vi "test - TMO of Sync-Reply.vi"(8 "error in (no error)":errorcluster, 11 "TestCase in":refnum<class "testcase-Basic-Function.lvclass">) -> (0 "error out":errorcluster, 3 "TestCase out":refnum<class "testcase-Basic-Function.lvclass">)   [LabVIEW 2017, in "testcase-Basic-Function.lvclass"]
uses:
  testcase-Basic-Function.lvclass
  src/user.lib/_NEVSTOP/Communicable State Machine(CSM)/AdvanceAPI/CSM - Revert Arguments-Safe String.vi
  src/user.lib/_NEVSTOP/Communicable State Machine(CSM)/AdvanceAPI/CSM - Make String Arguments Safe.vi
  src/user.lib/_NEVSTOP/Communicable State Machine(CSM)/AdvanceAPI/CSM - Break Down Multiple States String.vi
  src/user.lib/_NEVSTOP/Communicable State Machine(CSM)/AdvanceAPI/CSM - Compact Multiple States.vi
  src/user.lib/_NEVSTOP/Communicable State Machine(CSM)/AdvanceAPI/CSM - Keywords.vi
  src/user.lib/_NEVSTOP/Communicable State Machine(CSM)/_Shared/Trim Single-line Text.vi
  <vilib>/addons/_JKI Toolkits/VI Tester/TestCase.llb/TestCase.lvclass
  src/user.lib/_NEVSTOP/Communicable State Machine(CSM)/Communicable State Machine.lvlib
  C:/Program Files (x86)/National Instruments/LabVIEW 2017/vi.lib/addons/_JKI Toolkits/VI Tester/TestCase.llb/TestCase.lvclass
panel:
  out "x-y":u32
  out "State History":string
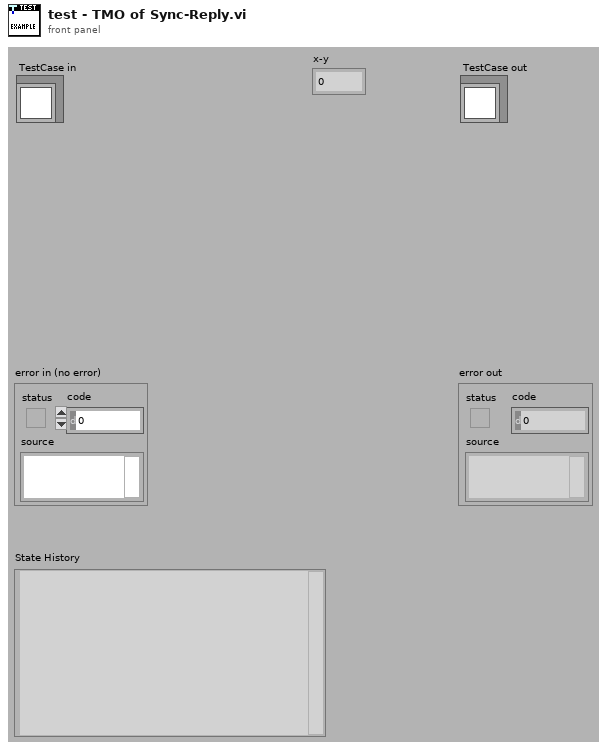
[diagram p1: front panel]
types:
  T1 = enum32{"Invalid", "Standard", "Closed", "Hidden", "Minimized", "Maximized"}
  T2 = enum32{"invalid app kind", "Development System", "Run Time System", "Student Edition", "Embedded LabVIEW", "Evaluation", "Custom"}
  T3 = typedef "Communicable State Machine.lvlib/_CSM_Response Source Message.ctl" = cluster{"‘State":string, "’Arguments":string, "’Error":errorcluster}
  T4 = cluster{"Current VI Reference":refnum<vi>, "Close Panel on Exit?":bool}
  T5 = cluster{"Core":cluster{"Current VI Reference":refnum<vi>, "Close Panel on Exit?":bool}, "Your Boolean data":bool, "Your string data":string}
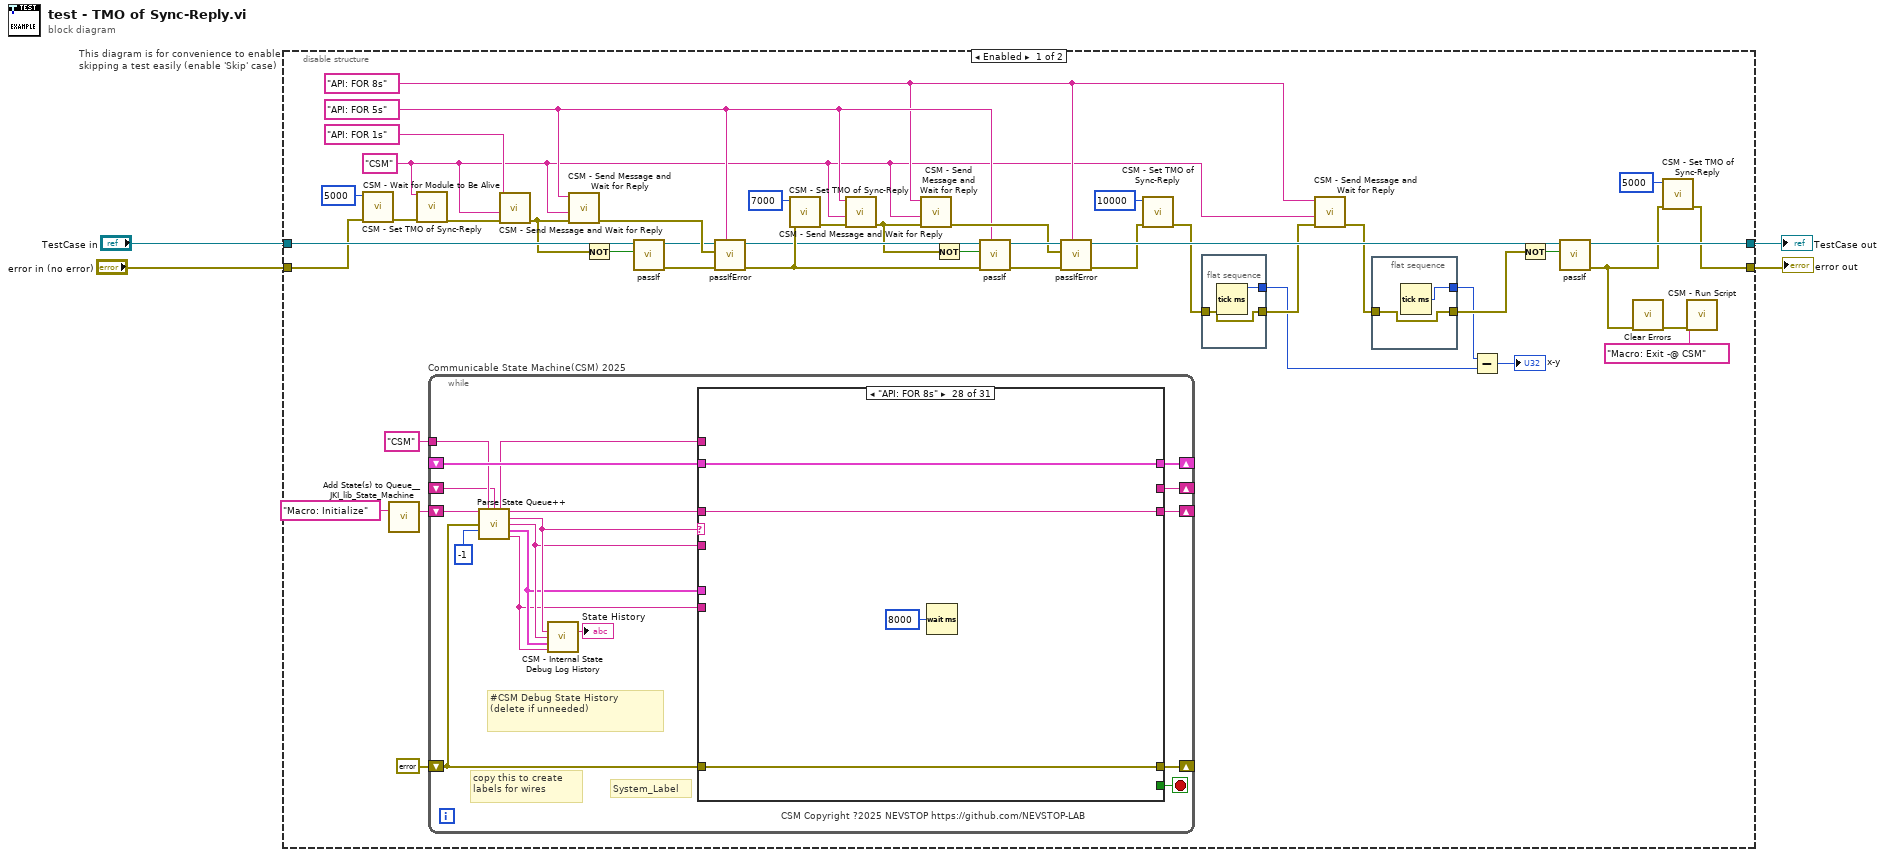
[diagram p0: block diagram]
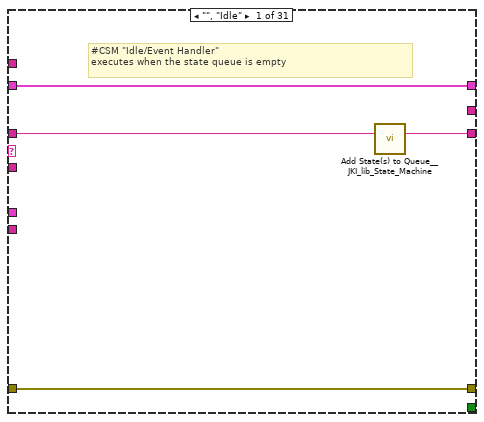
[diagram p2: hidden frame]
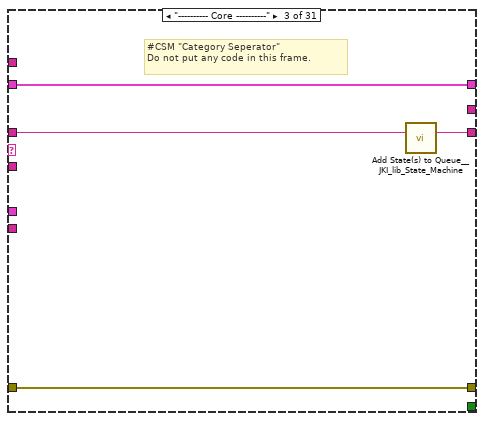
[diagram p4: hidden frame]
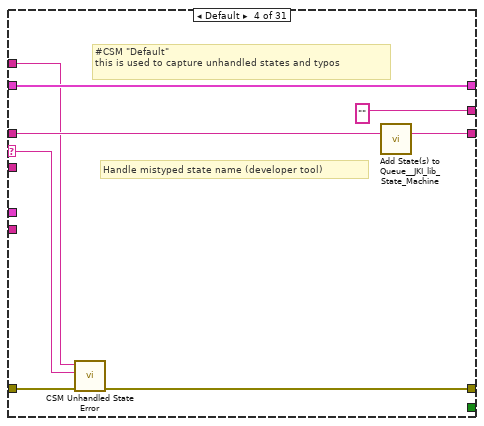
[diagram p5: hidden frame]
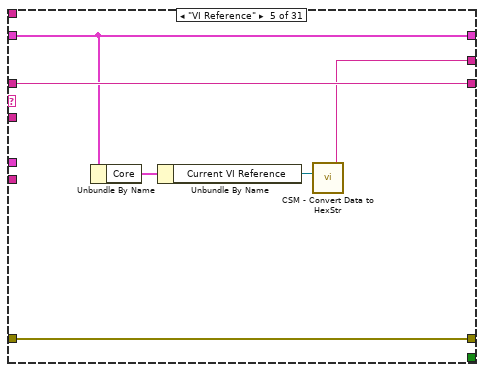
[diagram p6: hidden frame]
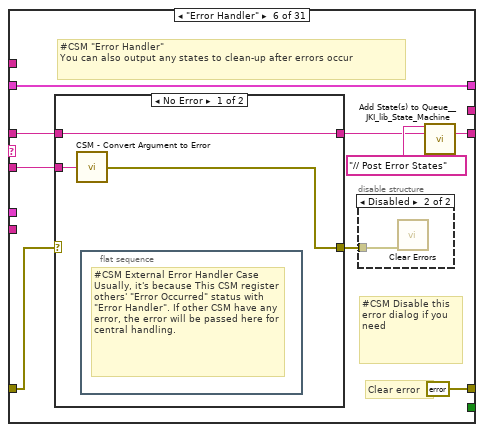
[diagram p7: hidden frame]
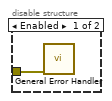
[diagram p8: hidden frame]
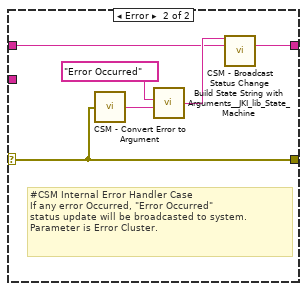
[diagram p9: hidden frame]
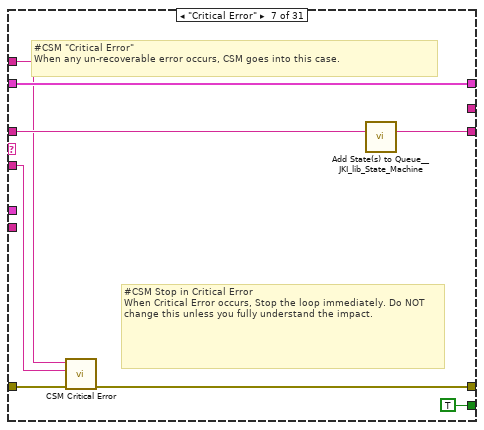
[diagram p10: hidden frame]
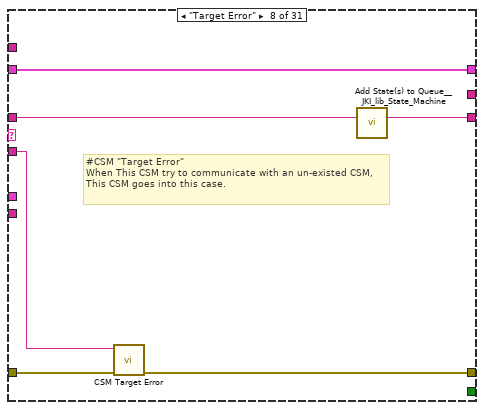
[diagram p11: hidden frame]
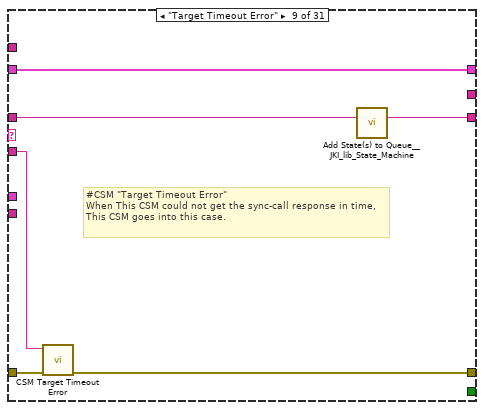
[diagram p12: hidden frame]
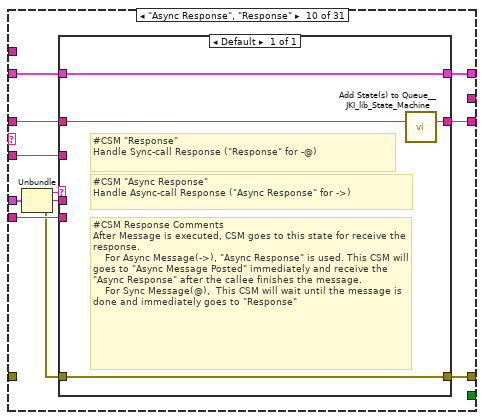
[diagram p13: hidden frame]
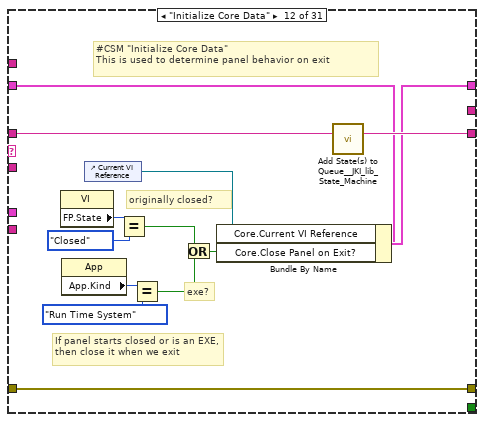
[diagram p15: hidden frame]
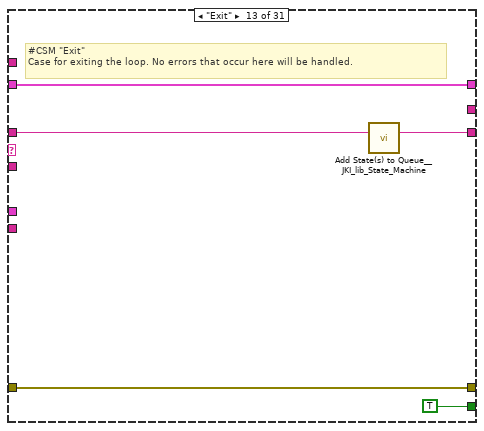
[diagram p16: hidden frame]
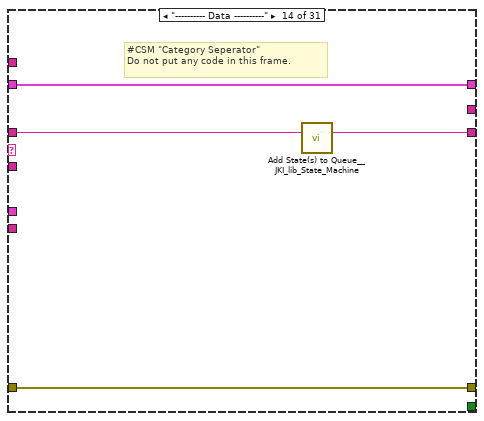
[diagram p17: hidden frame]
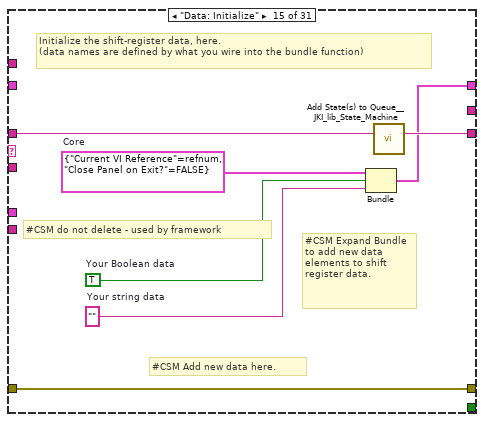
[diagram p18: hidden frame]
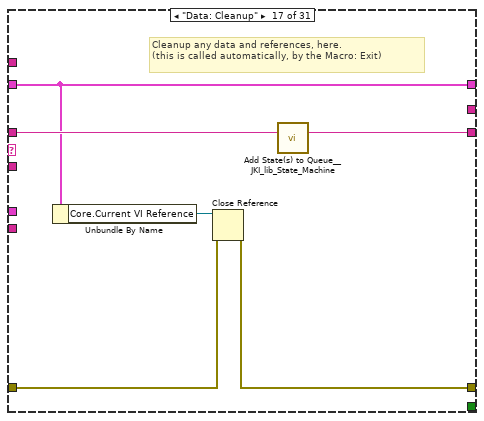
[diagram p20: hidden frame]
diagram:
  n1 = disable-structure "This diagram is for convenience to enable skipping a test easily (enable 'Skip' case)" shown="Enabled" {
    disable-tunnel: "TestCase in" -> [w40 w332]
    disable-tunnel: [w21 w330] -> w1
    disable-tunnel: [w5 w331] -> w3
    disable-tunnel: "error in (no error)" -> [w13 w329]
    frame Enabled {
      w23 = "API: FOR 8s" ("State")
      w27 = "API: FOR 5s" ("State")
      w18 = "CSM" ("Name (\"\" to Use UUID)")
      n2 = call "CSM - Set TMO of Sync-Reply.vi"("Error In"=w13, "TMO For Sync-Rep (Ms) In"=5000 ("TMO for Sync-Rep(ms)")) -> ("error out"=w14:errorcluster)  [unwired: 8 in, 1 out]
      n3 = call <vilib>:"Add State(s) to Queue__JKI_lib_State_Machine.vi"("State(s) in (\"\")"="Macro: Initialize" ("Init State(\"Macro: Initialize\")")) -> ("States Out"=w48:string)  [unwired: 14 in]
      n4 = call "CSM - Wait for Module to Be Alive.vi"("CSM Name"=w18, "error in (no error)"=w14) -> ("error out"=w44:errorcluster)  [unwired: 11 in, 2 out]
      n5 = while "Communicable State Machine(CSM) 2025" {
        shift-right: [w65] -> _
        shift-left: _ -> [w64]
        shift-right: [w68] -> _
        shift-left: errorcluster {"status"=FALSE, "code"=0, "source"=""} ("error out") -> [w63]
        shift-right: [w67] -> _
        shift-left: w48 -> [w69]
        tunnel: "CSM" ("Name (\"\" to Use UUID)") -> [w61]
        shift-right: [w62] -> _
        shift-left: _ -> [w55]
        stop <- w66 stop-if-true
        # "#CSM Debug State History\n(delete if unneeded)"
        # "copy this to create labels for wires"
        # "System_Label"
        # "CSM Copyright ?2025 NEVSTOP https://github.com/NEVSTOP-LAB"
        n6 = call "Parse State Queue++.vi"("State Queue"=w69, "Name (\"\" to Use UUID)"=w61, "Response Arguments"=w55, "Previous Error"=w63, "Dequeue Timeout (1 ms)"=-1 ("Timeout")) -> ("Name Used"=w56:string, "Remaining States"=w70:string, "Current State"=w60:string, "Arguments"=w59:string, ">> Response Source Message >>"=w58:T3, ">> Source CSM >>"=w57:string)  [unwired: 5 in]
        n7 = call "CSM - Internal State Debug Log History.vi"("State"=w60, "Arguments (\"\")"=w59, ">> Response Source Message >>"=w58, "Source (\"\")"=w57) -> ("Debug Log"=→"State History":string)  [unwired: 11 in]
        n8 = case shown="\"API: FOR 8s\"" w60 {
          selector: w60 -> [_ _ _ w84 _ _ _ _ _ _ _ _ _ _ _ _ _ _ _ _ _ _ _ _ _ _ _ _ _ _ _]
          tunnel: w70 -> [w71 w76 w81 w88 w94 w100 w121 w127 w133 w141 w152 w166 w171 w175 w182 w184 w191 w195 w199 w205 w220 w289 w294 w301 w303 w307 w311 w315 w320 w324 w328]
          tunnel: w59 -> [_ _ _ _ _ w99 w117 w126 w131 w140 _ _ _ _ _ _ _ _ _ w200 w214 _ _ _ _ _ _ _ _ _ _]
          tunnel: w64 -> [w72 w75 w78 w86 w93 w103 w122 w128 w134 w143 w151 w159 w169 w172 _ w183 w186 w192 w197 w203 w216 w286 w291 w298 w302 w306 w310 w314 w317 w321 w325]
          tunnel: [w73 w77 w79 w82 w95 errorcluster {"status"=FALSE, "code"=0, "source"=""} ("error out") w118 w124 w130 w146 w153 w163 w168 w173 w179 w185 w187 w193 w196 w201 w217 w287 w292 w299 w304 w308 w312 w316 w318 w322 w326] -> w68
          tunnel: w63 -> [w73 w77 w79 w89 w95 w101 w123 w125 w132 _ w153 w163 w168 w173 w179 w185 w188 w193 w196 w202 w218 w287 w292 w299 w304 w308 w312 w316 w318 w322 w326]
          tunnel: [w74 w76 w80 w87 w94 w96 w120 w129 w135 w142 w152 w165 w170 w174 w181 w184 w190 w194 w198 w204 w219 w288 w293 w300 w303 w307 w311 w315 w319 w323 w327] -> w67
          tunnel: [_ _ _ _ _ _ TRUE _ _ _ _ _ TRUE _ _ _ _ _ _ _ _ _ _ _ _ _ _ _ _ _ _] -> w66
          tunnel: [w72 w75 w78 w86 w93 w103 w122 w128 w134 w144 w151 w164 w169 w172 w180 w183 w186 w192 w197 w203 w216 w286 w291 w298 w302 w306 w310 w314 w317 w321 w325] -> w65
          tunnel: w57 -> [_ _ _ _ _ _ _ _ _ w138 _ _ _ _ _ _ _ _ _ _ _ _ _ _ _ _ _ _ _ _ _]
          tunnel: w58 -> [_ _ _ _ _ _ _ _ _ w145 _ _ _ _ _ _ _ _ _ _ _ _ _ _ _ _ _ _ _ _ _]
          tunnel: [_ _ _ "" w90 _ _ _ _ _ _ _ _ _ _ _ _ _ _ _ _ _ _ _ _ _ _ _ _ _ _] -> w62
          tunnel: w56 -> [_ _ _ w83 _ _ w116 _ _ _ _ _ _ _ _ _ _ _ _ _ _ _ _ _ _ _ _ _ _ _ _]
          frame "", "Idle" {
            # "#CSM \"Idle/Event Handler\"\nexecutes when the state queue is empty"
            n9 = call <vilib>:"Add State(s) to Queue__JKI_lib_State_Machine.vi"("State(s) in (\"\")"=w71) -> ("States Out"=w74:string)  [unwired: 14 in]
          }
          frame "CSM Documentation" {
            # "#CSM README FIRST\n\nCommunicable State Machine(CSM) is a LabVIEW application framework that builds upon JKI State Machine(JKISM). It follows the pattern of JKISM and extends the keywords to describe message communication between modules, including concepts such as Sync-Message, Async-Message, Subscription/Unsubscription of status - essential elements for creating reusable code modules. For more information, please visit the CSM wiki: https://nevstop-lab.github.io/CSM-Wiki/\n\nFor instructions on JKI State Machine, visit: http://jki.net/state-machine/\nFor information about CSM, visit: https://github.com/NEVSTOP-LAB"
            # "#CSM \"Documentation\"\nCase for holding CSM Documenation"
          }
          frame "---------- Core ----------" {
            # "#CSM \"Category Seperator\"\nDo not put any code in this frame."
            n10 = call <vilib>:"Add State(s) to Queue__JKI_lib_State_Machine.vi"("State(s) in (\"\")"=w81) -> ("States Out"=w80:string)  [unwired: 14 in]
          }
          frame Default {
            # "#CSM \"Default\"\nthis is used to capture unhandled states and typos"
            # "Handle mistyped state name (developer tool)"
            n11 = call "CSM Unhandled State Error.vi"("error in (no error)"=w89, "Current State"=w84, "CSM Name"=w83) -> ("error out"=w82:errorcluster)  [unwired: 8 in]
            n12 = call <vilib>:"Add State(s) to Queue__JKI_lib_State_Machine.vi"("State(s) in (\"\")"=w88) -> ("States Out"=w87:string)  [unwired: 14 in]
          }
          frame "VI Reference" {
            n13 = Unbundle By Name(w93) -> ("Core"=w92:T4)
            n14 = Unbundle By Name(w92) -> ("Current VI Reference"=w91:refnum<vi>)
            n15 = call "CSM - Convert Data to HexStr.vi"("Variant"=w91) -> ("HEX String (0-9,A-F)"=w90:string)  [unwired: 8 in]
          }
          frame "Error Handler" {
            # "#CSM Disable this error dialog if you need"
            # "#CSM \"Error Handler\"\nYou can also output any states to clean-up after errors occur"
            # "Clear error"
            n16 = case shown="No Error" w101 {
              selector: w101 -> [_ w110]
              tunnel: [w109 w112] -> w97
              tunnel: w100 -> [w109 w111]
              tunnel: w99 -> [w108 _]
              tunnel: [w107 w110] -> w102
              frame No Error {
                n17 = call "CSM - Convert Argument to Error.vi"("Argument"=w108) -> ("Error"=w107:errorcluster)  [unwired: 4 in]
                n18 = flat-sequence {
                  frame #0 {
                    # "#CSM External Error Handler Case\nUsually, it's because This CSM register others' \"Error Occurred\" status with \"Error Handler\". If other CSM have any error, the error will be passed here for central handling."
                  }
                }
              }
              frame Error {
                # "#CSM Internal Error Handler Case \nIf any error Occurred, \"Error Occurred\" \nstatus update will be broadcasted to system.\nParameter is Error Cluster."
                n19 = call "CSM - Convert Error to Argument.vi"("Error"=w110) -> ("Argument"=w114:string)  [unwired: 4 in]
                n20 = call <vilib>:"Build State String with Arguments__JKI_lib_State_Machine.vi"("Arguments (\"\")"=w114, "State"="Error Occurred" ("Status with Arguments")) -> ("State with Arguments"=w113:string)  [unwired: 4 in]
                n21 = call "CSM - Broadcast Status Change.vi"("Status With Arguments"=w113, "State Queue"=w111) -> ("Remaining States"=w112:string)  [unwired: 13 in]
              }
            }
            n22 = disable-structure shown="Disabled" {
              disable-tunnel: w102 -> [w105 w106]
              frame Enabled {
                n23 = call <vilib>:"General Error Handler.vi"("error in (no error)"=w105) -> ()  [unwired: 10 in, 5 out]
              }
              frame Disabled {
                n24 = call <vilib>:"Clear Errors.vi"("error in (no error)"=w106) -> ()  [unwired: 5 in, 2 out]
              }
            }
            n25 = call <vilib>:"Add State(s) to Queue__JKI_lib_State_Machine.vi"("State(s) in Front (\"\")"="// Post Error States", "State(s) in (\"\")"=w97) -> ("States Out"=w96:string)  [unwired: 13 in]
          }
          frame "Critical Error" {
            # "#CSM Stop in Critical Error\nWhen Critical Error occurs, Stop the loop immediately. Do NOT change this unless you fully understand the impact."
            # "#CSM \"Critical Error\"\nWhen any un-recoverable error occurs, CSM goes into this case."
            n26 = call "CSM Critical Error.vi"("error in (no error)"=w123, "Arugments (As Reason)"=w117, "CSM Name"=w116) -> ("error out"=w118:errorcluster)  [unwired: 8 in]
            n27 = call <vilib>:"Add State(s) to Queue__JKI_lib_State_Machine.vi"("State(s) in (\"\")"=w121) -> ("States Out"=w120:string)  [unwired: 14 in]
          }
          frame "Target Error" {
            # "#CSM \"Target Error\"\nWhen This CSM try to communicate with an un-existed CSM, This CSM goes into this case."
            n28 = call "CSM Target Error.vi"("error in (no error)"=w125, "Arguments (As CSM Name)"=w126) -> ("error out"=w124:errorcluster)  [unwired: 9 in]
            n29 = call <vilib>:"Add State(s) to Queue__JKI_lib_State_Machine.vi"("State(s) in (\"\")"=w127) -> ("States Out"=w129:string)  [unwired: 14 in]
          }
          frame "Target Timeout Error" {
            # "#CSM \"Target Timeout Error\"\nWhen This CSM could not get the sync-call response in time, This CSM goes into this case."
            n30 = call "CSM Target Timeout Error.vi"("error in (no error)"=w132, "Arguments (As CSM Name)"=w131) -> ("error out"=w130:errorcluster)  [unwired: 9 in]
            n31 = call <vilib>:"Add State(s) to Queue__JKI_lib_State_Machine.vi"("State(s) in (\"\")"=w133) -> ("States Out"=w135:string)  [unwired: 14 in]
          }
          frame "Async Response", "Response" {
            n32 = Unbundle(w145) -> ("‘State"=w139:string, "’Arguments"=w137:string, "’Error"=w136:errorcluster)
            n33 = case shown="Default" w139 {
              tunnel: [w150] -> w146
              tunnel: w136 -> [w150]
              tunnel: [w149] -> w144
              tunnel: w143 -> [w149]
              tunnel: [w147] -> w142
              tunnel: w141 -> [w148]
              tunnel: w140 -> [_]
              tunnel: w138 -> [_]
              tunnel: w137 -> [_]
              frame Default {
                # "#CSM Response Comments\nAfter Message is executed, CSM goes to this state for receive the response.\n    For Async Message(->), \"Async Response\" is used. This CSM will goes to \"Async Message Posted\" immediately and receive the \"Async Response\" after the callee finishes the message.\n    For Sync Message(@),  This CSM will wait until the message is done and immediately goes to \"Response\""
                # "#CSM \"Async Response\"\nHandle Async-call Response (\"Async Response\" for ->)"
                # "#CSM \"Response\"\nHandle Sync-call Response (\"Response\" for -@)"
                n34 = call <vilib>:"Add State(s) to Queue__JKI_lib_State_Machine.vi"("State(s) in (\"\")"=w148) -> ("States Out"=w147:string)  [unwired: 14 in]
              }
            }
          }
          frame "Async Message Posted" {
            # "#CSM \"Async Message Posted\"\nAfter Async Message is posted (-> or ->| ), CSM goes to this state for post-action.\nYou can use Argument - State to tell which Async Message is called."
          }
          frame "Initialize Core Data" {
            # "#CSM \"Initialize Core Data\"\nThis is used to determine panel behavior on exit"
            # "originally closed?"
            # "exe?"
            # "If panel starts closed or is an EXE, then close it when we exit"
            n35 = property class="VI"() -> ("FP.State"=w156:T1)  [unwired: 2 in, 2 out]
            n36 = property class="App"() -> ("App.Kind"=w162:T2)  [unwired: 2 in, 2 out]
            n37 = control-ref of="Current VI Reference"() -> (w157:refnum<vi>)
            n38 = Equal?(x=w156, y=T1."Closed" ("Front Panel Window:State")) -> (x = y?=w154:bool)
            n39 = Equal?(x=w162, y=T2."Run Time System" ("Application:Kind")) -> (x = y?=w160:bool)
            n40 = Or(x=w154, y=w160) -> (x .or. y?=w158:bool)
            n41 = Bundle By Name(cluster=w159, "Core.Current VI Reference"=w157, "Core.Close Panel on Exit?"=w158) -> (w164:T5)
            n42 = call <vilib>:"Add State(s) to Queue__JKI_lib_State_Machine.vi"("State(s) in (\"\")"=w166) -> ("States Out"=w165:string)  [unwired: 14 in]
          }
          frame "Exit" {
            # "#CSM \"Exit\"\nCase for exiting the loop. No errors that occur here will be handled."
            n43 = call <vilib>:"Add State(s) to Queue__JKI_lib_State_Machine.vi"("State(s) in (\"\")"=w171) -> ("States Out"=w170:string)  [unwired: 14 in]
          }
          frame "---------- Data ----------" {
            # "#CSM \"Category Seperator\"\nDo not put any code in this frame."
            n44 = call <vilib>:"Add State(s) to Queue__JKI_lib_State_Machine.vi"("State(s) in (\"\")"=w175) -> ("States Out"=w174:string)  [unwired: 14 in]
          }
          frame "Data: Initialize" {
            w176 = T4 {"Current VI Reference"=refnum, "Close Panel on Exit?"=FALSE}  # Core
            w178 = TRUE  # Your Boolean data
            w177 = ""  # Your string data
            # "#CSM do not delete - used by framework"
            # "#CSM Expand Bundle to add new data elements to shift register data."
            # "#CSM Add new data here."
            # "Initialize the shift-register data, here.\n(data names are defined by what you wire into the bundle function)"
            n45 = Bundle("Core"=w176, "Your Boolean data"=w178, "Your string data"=w177) -> (w180:T5)  [unwired: 1 in]
            n46 = call <vilib>:"Add State(s) to Queue__JKI_lib_State_Machine.vi"("State(s) in (\"\")"=w182) -> ("States Out"=w181:string)  [unwired: 14 in]
          }
          frame "Data: Update Indicators" {
          }
          frame "Data: Cleanup" {
            # "Cleanup any data and references, here.\n(this is called automatically, by the Macro: Exit)"
            n47 = Unbundle By Name(w186) -> ("Core.Current VI Reference"=w189:refnum<vi>)
            n48 = Close Reference(reference=w189, error in (no error)=w188) -> (error out=w187:errorcluster)
            n49 = call <vilib>:"Add State(s) to Queue__JKI_lib_State_Machine.vi"("State(s) in (\"\")"=w191) -> ("States Out"=w190:string)  [unwired: 14 in]
          }
          frame "---------- UI ----------" {
            # "#CSM \"Category Seperator\"\nDo not put any code in this frame."
            n50 = call <vilib>:"Add State(s) to Queue__JKI_lib_State_Machine.vi"("State(s) in (\"\")"=w195) -> ("States Out"=w194:string)  [unwired: 14 in]
          }
          frame "UI: Initialize" {
            # "#CSM \"UI: Initialize\"\nInitialize the User Interface, here.\n(this is called automatically, by the Macro: Init)"
            n51 = call <vilib>:"Add State(s) to Queue__JKI_lib_State_Machine.vi"("State(s) in (\"\")"=w199) -> ("States Out"=w198:string)  [unwired: 14 in]
          }
          frame "UI: Cursor Set" {
            # "#CSM \"UI: Cursor Set\"\nSet and Unset Cursor Busy.\n(Usage: \"UI: Cursor Set >> Busy|Idle\")"
            # "Argument"
            n52 = disable-structure shown="TARGET_TYPE!=Windows" {
              disable-tunnel: w202 -> [w208 w213]
              disable-tunnel: [w207 w213] -> w201
              disable-tunnel: w200 -> [w206 _]
              frame condition #0 (active) {
                n53 = case shown="\"Idle\", Default" w206 {
                  tunnel: w208 -> [w210 w212]
                  tunnel: [w209 w211] -> w207
                  frame "Idle", Default {
                    n54 = call <vilib>:"Unset Busy.vi"("error in (no error)"=w210) -> ("error out"=w209:errorcluster)  [unwired: 10 in]
                  }
                  frame "Busy" {
                    n55 = call <vilib>:"Set Busy.vi"("error in (no error)"=w212) -> ("error out"=w211:errorcluster)  [unwired: 9 in, 1 out]
                  }
                }
              }
              frame condition #1 {
              }
            }
            n56 = call <vilib>:"Add State(s) to Queue__JKI_lib_State_Machine.vi"("State(s) in (\"\")"=w205) -> ("States Out"=w204:string)  [unwired: 14 in]
          }
          frame "UI: Front Panel State" {
            # "#CSM \"UI: Front Panel State\"\nSet Front Panel Open or Closed\n(Usage: \"UI: Front Panel State >> Open|Close\")"
            # "Argument"
            n57 = Unbundle By Name(w216) -> ("Core.Current VI Reference"=w215:refnum<vi>)
            n58 = call <vilib>:"Add State(s) to Queue__JKI_lib_State_Machine.vi"("State(s) in (\"\")"=w220) -> ("States Out"=w219:string)  [unwired: 14 in]
            n59 = case shown="\"Close\", \"Closed\"" w214 {
              tunnel: w218 -> [w226 w241 w252 w265 w278]
              tunnel: [w228 w242 w254 w267 w280] -> w217
              tunnel: w215 -> [w227 w239 w253 w266 w279]
              frame "Open", "Standard", Default {
                w221 = T1."Standard" ("State")
                n60 = property class="VI"(reference=w227, error in=w226) -> (reference out=w224:refnum<vi>, error out=w225:errorcluster, "FP.State"=w223:T1)
                n61 = Not Equal?(x=w223, y=w221) -> (x != y?=w222:bool)
                n62 = case shown="True" w222 {
                  tunnel: [w232 w234] -> w228
                  tunnel: w225 -> [w231 w234]
                  tunnel: w224 -> [w230 _]
                  tunnel: w221 -> [w229 _]
                  frame True {
                    n63 = invoke class="VI" method="FP.Open"(reference=w230, error in=w231, "Activate"=TRUE, "State"=w229) -> (error out=w232:errorcluster)  [unwired: 1 in, 4 out]
                  }
                  frame False {
                  }
                }
              }
              frame "Close", "Closed" {
                n64 = property class="VI"(reference=w239, error in=w241) -> (reference out=w238:refnum<vi>, error out=w240:errorcluster, "FP.State"=w236:T1)
                n65 = Not Equal?(x=w236, y=T1."Closed" ("Front Panel Window:State")) -> (x != y?=w235:bool)
                n66 = case shown="False" w235 {
                  tunnel: [w243 w246] -> w242
                  tunnel: w240 -> [w243 w245]
                  tunnel: w238 -> [_ w244]
                  frame False {
                  }
                  frame True {
                    n67 = invoke class="VI" method="FP.Close"(reference=w244, error in=w245) -> (error out=w246:errorcluster)  [unwired: 1 in, 2 out]
                  }
                }
              }
              frame "Hidden", "Hide" {
                w247 = T1."Hidden" ("State")
                n68 = property class="VI"(reference=w253, error in=w252) -> (reference out=w250:refnum<vi>, error out=w251:errorcluster, "FP.State"=w249:T1)
                n69 = Not Equal?(x=w249, y=w247) -> (x != y?=w248:bool)
                n70 = case shown="True" w248 {
                  tunnel: [w258 w259] -> w254
                  tunnel: w251 -> [w257 w259]
                  tunnel: w250 -> [w256 _]
                  tunnel: w247 -> [w255 _]
                  frame True {
                    n71 = invoke class="VI" method="FP.Open"(reference=w256, error in=w257, "State"=w255) -> (error out=w258:errorcluster)  [unwired: 2 in, 4 out]
                  }
                  frame False {
                  }
                }
              }
              frame "Minimize", "Minimized" {
                w260 = T1."Minimized" ("State")
                n72 = property class="VI"(reference=w266, error in=w265) -> (reference out=w263:refnum<vi>, error out=w264:errorcluster, "FP.State"=w262:T1)
                n73 = Not Equal?(x=w262, y=w260) -> (x != y?=w261:bool)
                n74 = case shown="True" w261 {
                  tunnel: [w271 w272] -> w267
                  tunnel: w264 -> [w270 w272]
                  tunnel: w263 -> [w269 _]
                  tunnel: w260 -> [w268 _]
                  frame True {
                    n75 = invoke class="VI" method="FP.Open"(reference=w269, error in=w270, "State"=w268) -> (error out=w271:errorcluster)  [unwired: 2 in, 4 out]
                  }
                  frame False {
                  }
                }
              }
              frame "Maximize", "Maximized" {
                w273 = T1."Maximized" ("State")
                n76 = property class="VI"(reference=w279, error in=w278) -> (reference out=w276:refnum<vi>, error out=w277:errorcluster, "FP.State"=w275:T1)
                n77 = Not Equal?(x=w275, y=w273) -> (x != y?=w274:bool)
                n78 = case shown="True" w274 {
                  tunnel: [w284 w285] -> w280
                  tunnel: w277 -> [w283 w285]
                  tunnel: w276 -> [w282 _]
                  tunnel: w273 -> [w281 _]
                  frame True {
                    n79 = invoke class="VI" method="FP.Open"(reference=w282, error in=w283, "State"=w281) -> (error out=w284:errorcluster)  [unwired: 2 in, 4 out]
                  }
                  frame False {
                  }
                }
              }
            }
          }
          frame "---------- Macro ----------" {
            # "#CSM \"Category Seperator\"\nDo not put any code in this frame."
            n80 = call <vilib>:"Add State(s) to Queue__JKI_lib_State_Machine.vi"("State(s) in (\"\")"=w289) -> ("States Out"=w288:string)  [unwired: 14 in]
          }
          frame "Macro: Initialize" {
            # "#CSM \"Macro: Initialize\"\nInitialization Macro (This is called once, when the VI starts)"
            n81 = call <vilib>:"Add State(s) to Queue__JKI_lib_State_Machine.vi"("State(s) in Front (\"\")"="Data: Initialize\nInitialize Core Data\nData: Update Indicators", "State(s) in (\"\")"=w294) -> ("States Out"=w293:string)  [unwired: 13 in]
          }
          frame "Macro: Exit" {
            # "#CSM \"Macro: Exit\"\nExit Macro (This is called once, when the VI exits)"
            n82 = call <vilib>:"Add State(s) to Queue__JKI_lib_State_Machine.vi"("State(s) in Front (\"\")"="//Exit Sub-Modules ", "State(s) at Back (\"\")"="Data: Cleanup\nExit") -> ("States Out"=w296:string)  [unwired: 13 in]
            n83 = call <vilib>:"Add State(s) to Queue__JKI_lib_State_Machine.vi"("State(s) in Front (\"\")"=w296, "State(s) in (\"\")"=w301) -> ("States Out"=w300:string)  [unwired: 13 in]
          }
          frame "---------- API ----------" {
            # "#CSM \"Category Seperator\"\nDo not put any code in this frame."
          }
          frame "API: FOR 5s" {
            n84 = Wait (ms)(milliseconds to wait=u32 5000) -> ()  [unwired: 1 out]
          }
          frame "API: FOR 1s" {
            n85 = Wait (ms)(milliseconds to wait=u32 1000) -> ()  [unwired: 1 out]
          }
          frame "API: FOR 8s" {
            n86 = Wait (ms)(milliseconds to wait=u32 8000) -> ()  [unwired: 1 out]
          }
          frame "---------- Action ----------" {
            # "#CSM \"Category Seperator\"\nDo not put any code in this frame."
            n87 = call <vilib>:"Add State(s) to Queue__JKI_lib_State_Machine.vi"("State(s) in (\"\")"=w320) -> ("States Out"=w319:string)  [unwired: 14 in]
          }
          frame "Action: action1" {
            # "#CSM \"Internal State\"\nThis category is used for holding internal states"
            n88 = call <vilib>:"Add State(s) to Queue__JKI_lib_State_Machine.vi"("State(s) in (\"\")"=w324) -> ("States Out"=w323:string)  [unwired: 14 in]
          }
          frame "Action: action2" {
            # "#CSM \"Internal State\"\nThis category is used for holding internal states"
            n89 = call <vilib>:"Add State(s) to Queue__JKI_lib_State_Machine.vi"("State(s) in (\"\")"=w328) -> ("States Out"=w327:string)  [unwired: 14 in]
          }
        }
      }
      n90 = call "CSM - Send Message and Wait for Reply.vi"("Error In (No Error)"=w44, "Target Module"=w18, "State"="API: FOR 1s") -> ("error out"=w16:errorcluster)  [unwired: 6 in, 2 out]
      n91 = call "CSM - Send Message and Wait for Reply.vi"("Error In (No Error)"=w16, "Target Module"=w18, "State"=w27) -> ("error out"=w42:errorcluster)  [unwired: 6 in, 2 out]
      n92 = Not(x=w16) -> (.not. x?=w41:bool)
      n93 = call-dynamic "passIf.vi"("pass"=w41, "TestCase in"=w40) -> ("error out"=w38:errorcluster, "TestCase out"=w39:refnum<class "testcase-Basic-Function.lvclass">)  [unwired: 8 in]
      n94 = call-dynamic "passIfError.vi"("custom report message (\"\")"=w27, "error in (no error)"=w38, "error"=w42, "TestCase in"=w39) -> ("error out"=w31:errorcluster, "TestCase out"=w30:refnum<class "testcase-Basic-Function.lvclass">)  [unwired: 6 in]
      n95 = call "CSM - Set TMO of Sync-Reply.vi"("Error In"=w31, "TMO For Sync-Rep (Ms) In"=7000 ("TMO for Sync-Rep(ms)")) -> ("error out"=w32:errorcluster)  [unwired: 8 in, 1 out]
      n96 = call "CSM - Send Message and Wait for Reply.vi"("Error In (No Error)"=w32, "Target Module"=w18, "State"=w27) -> ("error out"=w17:errorcluster)  [unwired: 6 in, 2 out]
      n97 = call "CSM - Send Message and Wait for Reply.vi"("Error In (No Error)"=w17, "Target Module"=w18, "State"=w23) -> ("error out"=w33:errorcluster)  [unwired: 6 in, 2 out]
      n98 = Not(x=w17) -> (.not. x?=w34:bool)
      n99 = call-dynamic "passIf.vi"("custom report message (\"\")"=w27, "error in (no error)"=w31, "pass"=w34, "TestCase in"=w30) -> ("error out"=w36:errorcluster, "TestCase out"=w35:refnum<class "testcase-Basic-Function.lvclass">)  [unwired: 6 in]
      n100 = call-dynamic "passIfError.vi"("custom report message (\"\")"=w23, "error in (no error)"=w36, "error"=w33, "TestCase in"=w35) -> ("error out"=w25:errorcluster, "TestCase out"=w26:refnum<class "testcase-Basic-Function.lvclass">)  [unwired: 6 in]
      n101 = call "CSM - Set TMO of Sync-Reply.vi"("Error In"=w25, "TMO For Sync-Rep (Ms) In"=10000 ("TMO for Sync-Rep(ms)")) -> ("error out"=w24:errorcluster)  [unwired: 8 in, 1 out]
      n102 = flat-sequence {
        tunnel: w24 -> [w51]
        tunnel: [w51] -> w12
        tunnel: [w52] -> w9
        frame #0 {
          n103 = Tick Count (ms)() -> (millisecond timer value=w52:u32)
        }
      }
      n104 = call "CSM - Send Message and Wait for Reply.vi"("Error In (No Error)"=w12, "Target Module"=w18, "State"=w23) -> ("error out"=w22:errorcluster)  [unwired: 6 in, 2 out]
      n105 = flat-sequence {
        tunnel: w22 -> [w49]
        tunnel: [w49] -> w11
        tunnel: [w50] -> w10
        frame #0 {
          n106 = Tick Count (ms)() -> (millisecond timer value=w50:u32)
        }
      }
      n107 = Subtract(x=w10, y=w9) -> (x-y=→"x-y":u32)
      n108 = Not(x=w11) -> (.not. x?=w28:bool)
      n109 = call-dynamic "passIf.vi"("pass"=w28, "TestCase in"=w26) -> ("error out"=w6:errorcluster, "TestCase out"=w21:refnum<class "testcase-Basic-Function.lvclass">)  [unwired: 8 in]
      n110 = call <vilib>:"Clear Errors.vi"("error in (no error)"=w6) -> ("error out"=w20:errorcluster)  [unwired: 5 in, 1 out]
      n111 = call "CSM - Set TMO of Sync-Reply.vi"("Error In"=w6, "TMO For Sync-Rep (Ms) In"=5000 ("TMO for Sync-Rep(ms) In")) -> ("error out"=w5:errorcluster)  [unwired: 8 in, 1 out]
      n112 = call "CSM - Run Script.vi"("CSM Scripts"="Macro: Exit -@ CSM", "error in (no error)"=w20) -> ()  [unwired: 11 in, 3 out]
    }
    frame Disabled {
      # "skip test result while test is under development"
      n113 = call <vilib>:"skip.vi"("error in (no error)"=w329, "TestCase in"=w332) -> ("error out"=w331:errorcluster, "TestCase out"=w330:refnum<class "testcase-Basic-Function.lvclass">)  [unwired: 8 in]
    }
  }
  "error out" <- w3
  "TestCase out" <- w1
